vi "Heat_Exch_Guide-plot.vi"(6 "Time In":i32, 8 "Temperature Sync":i32, 9 "Temp Band % (e.g. 1%=1.01)":dbl=1.04, 10 "Mean(Off)/Interval(On)":bool, 11 "TempGuide":bool) -> (0 "Graph 4":dbl, 1 "Graph 3":dbl, 2 "Graph 2":dbl, 3 "Graph 1":dbl, 4 "Time out":i32)   [LabVIEW 2014]
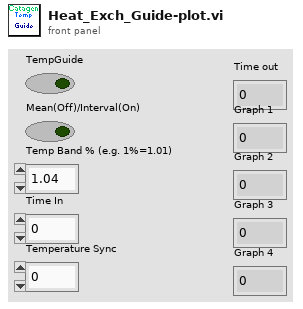
[diagram p1: front panel]
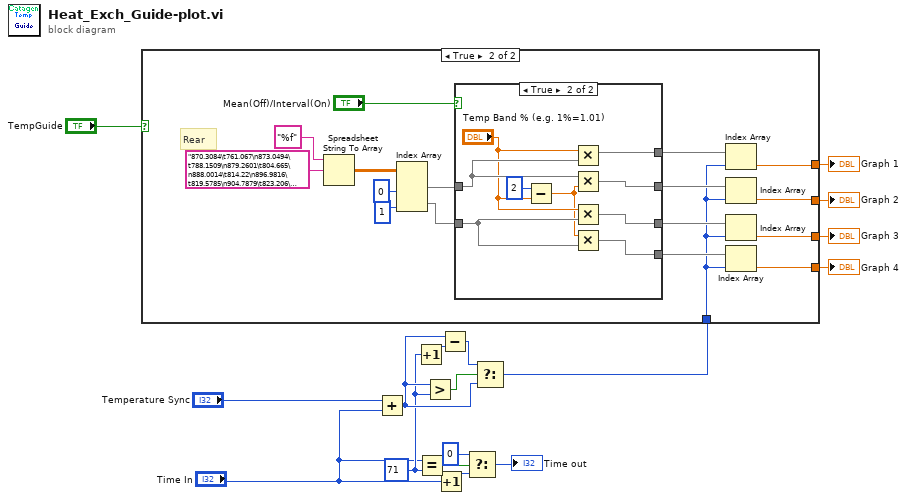
[diagram p0: block diagram]
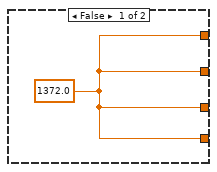
[diagram p2: hidden frame]
diagram:
  w8 = 71 ("y")
  n1 = Add(x="Temperature Sync", y="Time In") -> (x+y=w10:i32)
  n2 = Increment(x=w8) -> (x+1=w9:i32)
  n3 = Equal?(x="Time In", y=w8) -> (x = y?=w15:bool)
  n4 = Greater?(x=w10, y=w8) -> (0:w12:bool)
  n5 = Increment(x="Time In") -> (x+1=w13:i32)
  n6 = Subtract(x=w10, y=w9) -> (x-y=w11:i32)
  n7 = Select(t=0, s=w15, f=w13) -> (s? t:f=→"Time out":i32)
  n8 = Select(t=w11, s=w12, f=w10) -> (s? t:f=w7:i32)
  n9 = case shown="True" "TempGuide" {
    tunnel: w7 -> [_ w24]
    tunnel: [w18 w20] -> w4
    tunnel: [w18 w21] -> w3
    tunnel: [w18 w23] -> w2
    tunnel: [w18 w22] -> w1
    frame False {
      w18 = 1372.0
    }
    frame True {
      # "Rear"
      n10 = Spreadsheet String To Array(format string="%f", spreadsheet string="870.3084\t761.067\n873.0494\t788.1509\n879.2601\t804.665\n888.0014\t814.22\n896.9816\t819.5785\n904.7879\t823.206\n911.9924\t824.7308\n917.6064\t825.0215\n921.6508\t825.1518\n924.821\t825.413\n927.0153\t825.7409\n928.5058\t826.1208\n929.6235\t826.4765\n930.4462\t826.8204\n931.0392\t827.1783\n931.5569\t827.5233\n931.9779\t827.8205\n932.3272\t828.105\n932.6625\t828.3385\n932.9575\t828.6134\n933.2111\t828.8335\n933.4719\t829.092\n933.7198\t829.4003\n933.8864\t829.6565\n934.0886\t829.8649\n934.3606\t830.0872\n934.5106\t828.9752\n934.5648\t815.4966\n934.4297\t760.1573\n934.0106\t690.3177\n933.0675\t639.8207\n926.5606\t601.801\n911.8949\t571.4993\n893.9394\t561.1847\n880.8663\t627.0161\n875.4098\t721.9481\n878.2422\t778.466\n886.0113\t808.265\n894.1225\t820.6809\n901.9893\t822.1631\n908.3996\t823.212\n913.3358\t824.4128\n917.7932\t825.3224\n921.5556\t825.9809\n924.6686\t826.5365\n927.4009\t826.9582\n929.4949\t827.3705\n930.9829\t827.7757\n932.1224\t828.1188\n932.8592\t828.4355\n933.3227\t828.7444\n933.6686\t829.0765\n933.9301\t829.3471\n934.1551\t829.627\n934.382\t829.868\n934.6243\t830.1034\n934.8474\t830.3397\n935.0842\t830.5899\n935.313\t830.8214\n935.4586\t831.0425\n935.7013\t831.2267\n935.9896\t831.4431\n936.1238\t829.6628\n936.1419\t813.5719\n935.9612\t753.6579\n935.5023\t685.2665\n934.5043\t636.8912\n928.9561\t599.3783\n916.584\t569.9742\n899.2455\t559.9563\n883.0217\t625.8916\n873.3305\t712.123") -> (array=w34:dbl[][])  [unwired: 2 in]
      n11 = Index Array(array=w34, index (col) #1=0 ("disabled index (col)"), index (col) #2=1 ("disabled index (col)")) -> (element #1=w31:dbl[], element #2=w30:dbl[])  [unwired: 2 in]
      n12 = case shown="True" "Mean(Off)/Interval(On)" {
        tunnel: w31 -> [w36 w43]
        tunnel: w30 -> [w37 w40]
        tunnel: [w37 w38] -> w29
        tunnel: [w37 w42] -> w28
        tunnel: [w36 w44] -> w26
        tunnel: [w36 w45] -> w25
        frame False {
        }
        frame True {
          n13 = Subtract(x=2, y="Temp Band % (e.g. 1%=1.01)") -> (x-y=w39:dbl)
          n14 = Multiply(x="Temp Band % (e.g. 1%=1.01)", y=w43) -> (x*y=w45:dbl[])
          n15 = Multiply(x=w43, y=w39) -> (x*y=w44:dbl[])
          n16 = Multiply(x="Temp Band % (e.g. 1%=1.01)", y=w40) -> (x*y=w38:dbl[])
          n17 = Multiply(x=w39, y=w40) -> (x*y=w42:dbl[])
        }
      }
      n18 = Index Array(array=w25, index=w24) -> (element=w20:dbl)
      n19 = Index Array(array=w26, index=w24) -> (element=w21:dbl)
      n20 = Index Array(array=w29, index=w24) -> (element=w23:dbl)
      n21 = Index Array(array=w28, index=w24) -> (element=w22:dbl)
    }
  }
  "Graph 1" <- w4
  "Graph 2" <- w3
  "Graph 3" <- w2
  "Graph 4" <- w1
